vi "list.vi"(0 "error in (no error)":errorcluster) -> (1 "error out":errorcluster, 2 "serialList":string, 3 "return":i32)   [LabVIEW 2013, in "EM_CVx.lvlib"]
uses:
  EM_CVx.lvlib
  library/moverLibrary_x64.dll
  library/moverLibrary_x86.dll
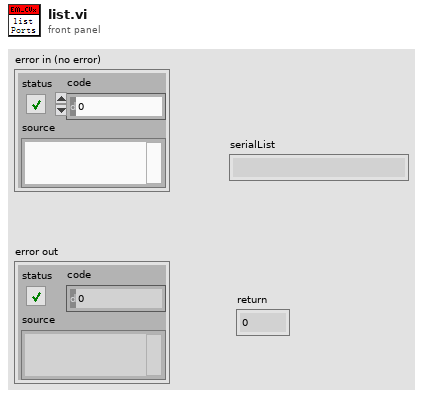
[diagram p1: front panel]
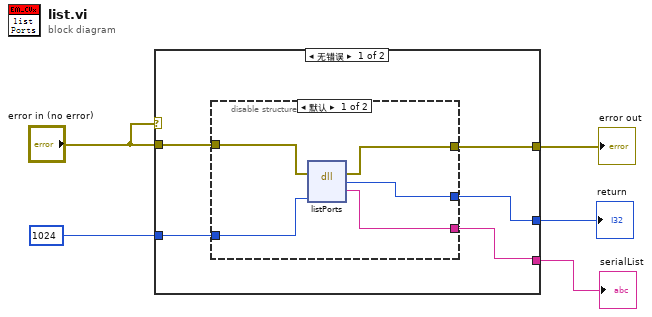
[diagram p0: block diagram]
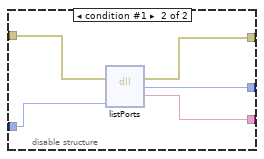
[diagram p2: hidden frame]
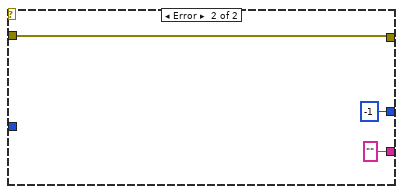
[diagram p3: hidden frame]
diagram:
  n1 = case shown="无错误" "error in (no error)" {
    tunnel: "error in (no error)" -> [w10 w23]
    tunnel: [w9 w23] -> w4
    tunnel: [w8 -1 ("return")] -> w3
    tunnel: 1024 ("length") -> [w7 _]
    tunnel: [w6 "" ("serialName")] -> w1
    frame No Error {
      n2 = disable-structure shown="默认" {
        disable-tunnel: w10 -> [w15 w20]
        disable-tunnel: [w14 w19] -> w9
        disable-tunnel: [w13 w18] -> w8
        disable-tunnel: w7 -> [w12 w17]
        disable-tunnel: [w11 w16] -> w6
        frame condition #0 (active) {
          n3 = dll-call lib="E:/5-mover/4-labView/EM_CVx_2013/library/moverLibrary_x86.dll" fn="listPorts"(error in=w15, "length"=w12) -> (error out=w14:errorcluster, "return"=w13:i32, "serialName"=w11:string)  [unwired: 4 in, 1 out]
        }
        frame condition #1 {
          n4 = dll-call lib="E:/5-mover/4-labView/EM_CVx_2013/library/moverLibrary_x64.dll" fn="listPorts"(error in=w20, "length"=w17) -> (error out=w19:errorcluster, "return"=w18:i32, "serialName"=w16:string)  [unwired: 4 in, 1 out]
        }
      }
    }
    frame Error {
    }
  }
  "error out" <- w4
  "return" <- w3
  "serialList" <- w1
